vi "Decide next action (polarization-based).vi"(8 "error in (no error)":errorcluster, 10 "Seek positive polarization?":bool, 11 "Automatic Mode in":refnum<class "Automatic Mode.lvclass">) -> (0 "error out":errorcluster, 1 "Should reseek?":bool, 2 "Decision":T1, 3 "Automatic Mode out":refnum<class "Automatic Mode.lvclass">)   [LabVIEW 2018, in "Automatic Mode.lvclass"]
uses:
  Automatic Mode.lvclass
  Controller decision.ctl
  Automatic Mode.lvclass/Automatic Mode.ctl
  <vilib>/Analysis/baseanly.llb/Mean (DBL).vi
  <vilib>/gmath/NI_Gmath.lvlib
  <vilib>/Analysis/NI_AALBase.lvlib
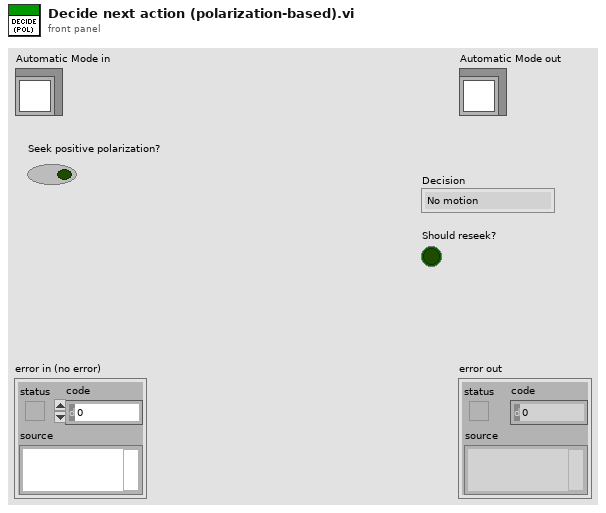
[diagram p1: front panel]
types:
  T1 = typedef "Controller decision.ctl" = enum16{"No motion", "Switch direction", "Keep current direction"}
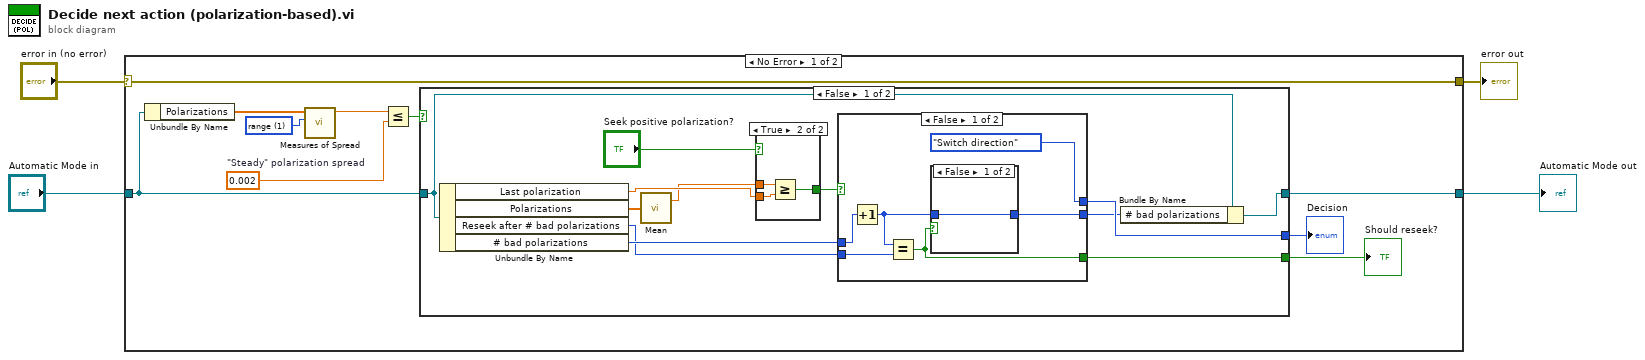
[diagram p0: block diagram]
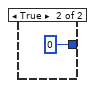
[diagram p2: hidden frame]
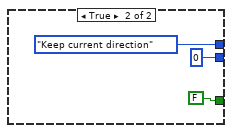
[diagram p3: hidden frame]
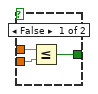
[diagram p4: hidden frame]
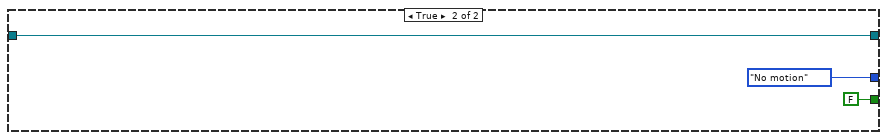
[diagram p5: hidden frame]
diagram:
  n1 = case shown="No Error" "error in (no error)" {
    selector: "error in (no error)" -> [w14 w48]
    tunnel: [w14 w48] -> w3
    tunnel: [w13 w47] -> w1
    tunnel: "Automatic Mode in" -> [w11 w47]
    frame No Error {
      w6 = 0.002  # "Steady" polarization spread
      w10 = 1 items=["standard deviation", "range", "mean absolute deviation", "interquartile range"] ("type")
      n2 = Unbundle By Name(w11) -> ("Polarizations"=w9:dbl[])
      n3 = call <vilib>:"Measures of Spread.vi"("type"=w10, "x array"=w9) -> ("spread value"=w8:dbl)  [unwired: 8 in, 1 out]
      n4 = Less Or Equal?(x=w8, y=w6) -> (x <= y?=w7:bool)
      n5 = case shown="False" w7 {
        tunnel: [w16 w45] -> w13
        tunnel: [w23 Controller_decision."No motion" ("Decision")] -> w12
        tunnel: w11 -> [w20 w45]
        tunnel: [w17 FALSE] -> w5
        frame False {
          n6 = Unbundle By Name(w20) -> ("Last polarization"=w25:dbl, "Polarizations"=w22:dbl[], "Reseek after # bad polarizations"=w15:u32, "# bad polarizations"=w18:u32)
          n7 = call-poly <vilib>:"Mean.vi"("X"=w22) -> ("mean"=w21:dbl)  [unwired: 1 out]
          n8 = case shown="True" "Seek positive polarization?" {
            tunnel: w21 -> [w40 w43]
            tunnel: w25 -> [w39 w42]
            tunnel: [w38 w41] -> w24
            frame False {
              n9 = Less Or Equal?(x=w40, y=w39) -> (x <= y?=w38:bool)
            }
            frame True {
              n10 = Greater Or Equal?(x=w43, y=w42) -> (x >= y?=w41:bool)
            }
          }
          n11 = case shown="False" w24 {
            tunnel: [Controller_decision."Switch direction" ("Decision") Controller_decision."Keep current direction" ("Decision")] -> w23
            tunnel: [w28 u32 0] -> w19
            tunnel: w18 -> [w31 _]
            tunnel: [w29 FALSE] -> w17
            tunnel: w15 -> [w30 _]
            frame False {
              n12 = Increment(x=w31) -> (x+1=w27:u32)
              n13 = Equal?(x=w27, y=w30) -> (x = y?=w29:bool)
              n14 = case shown="False" w29 {
                tunnel: [w33 0] -> w28
                tunnel: w27 -> [w33 _]
                frame False {
                }
                frame True {
                }
              }
            }
            frame True {
            }
          }
          n15 = Bundle By Name(cluster=w20, "# bad polarizations"=w19) -> (w16:refnum<class "Automatic Mode.lvclass">)
        }
        frame True {
        }
      }
      "Decision" <- w12
      "Should reseek?" <- w5
    }
    frame Error {
    }
  }
  "error out" <- w3
  "Automatic Mode out" <- w1
